vi "RT是否发送全局.vi"() -> ()   [LabVIEW 2013]
panel:
  out "是否发送数据":bool
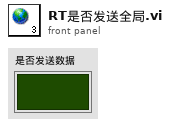
[diagram p1: front panel]
diagram:
